vi "DataCell_NbPASSFAIL_Bool.vi"(11 "Tableau en entrée":bool[](array[boolean])) -> (1 "Chaîne":string, 2 "Chaîne 2":string, 3 "Tableau en sortie":string[](array[string]))   [LabVIEW 2020]
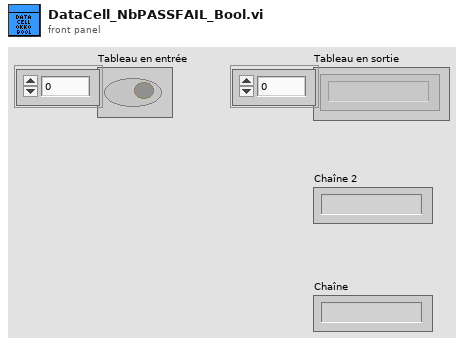
[diagram p1: front panel]
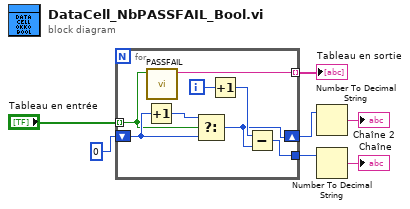
[diagram p0: block diagram]
diagram:
  n1 = for {
    tunnel: "Tableau en entrée" -> [w8] mode=indexing
    tunnel: [w9] -> w7 mode=indexing
    shift-right: [w11] -> w3
    shift-left: 0 -> [w14]
    tunnel: [w10] -> w4
    i -> [w13]
    n2 = Increment(x=w14) -> (x+1=w15:i32)
    n3 = call "PASSFAIL.vi"("E"=w8) -> ("S"=w9:string)  [unwired: 10 in]
    n4 = Select(t=w15, s=w8, f=w14) -> (s? t:f=w11:i32)
    n5 = Increment(x=w13) -> (x+1=w12:i32)
    n6 = Subtract(x=w12, y=w11) -> (x-y=w10:i32)
  }
  "Tableau en sortie" <- w7
  n7 = Number To Decimal String(number=w3) -> (decimal integer string=→"Chaîne 2":string)  [unwired: 1 in]
  n8 = Number To Decimal String(number=w4) -> (decimal integer string=→"Chaîne":string)  [unwired: 1 in]
